vi "GetTimeout.vi"(8 "error in":errorcluster, 10 "ArgIndex(0)":i32, 11 "Args":string[](array[string])) -> (0 "error out":errorcluster, 2 "TimeoutString":string, 3 "Timeout(Sec)":i32)   [LabVIEW 2020]
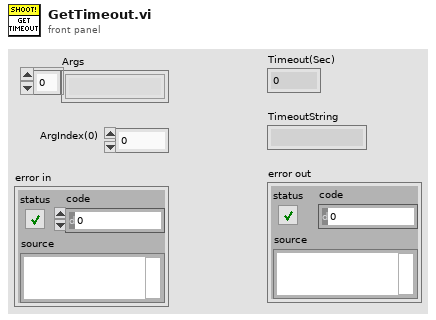
[diagram p1: front panel]
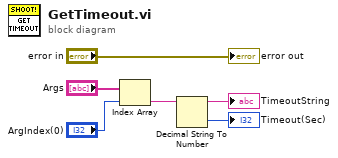
[diagram p0: block diagram]
diagram:
  n1 = Index Array(array="Args", index="ArgIndex(0)") -> (element=w3:string)
  "TimeoutString" <- w3
  n2 = Decimal String To Number(string=w3) -> (number=→"Timeout(Sec)":i32)  [unwired: 2 in, 1 out]
  "error out" <- "error in"
